vi "AG34980A Get Scan List.vi"(0 "VISA resource name":refnum<visa-resource-name>, 11 "error in (no error)":errorcluster) -> (4 "Channel List":string, 6 "Num of Chans":i32, 15 "error out":errorcluster)   [LabVIEW 2016]
doc: "This VI can be used to query the current scan list size as well as the time that the current scan started."
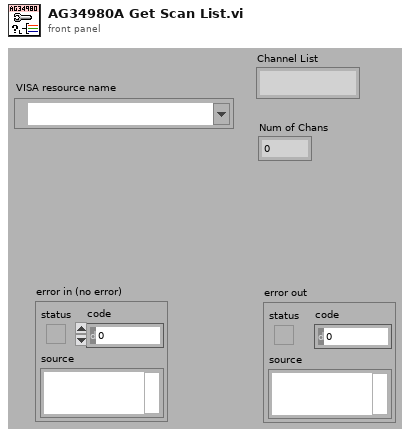
[diagram p1: front panel]
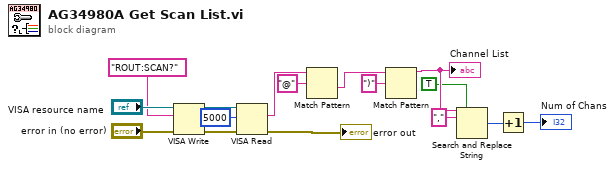
[diagram p0: block diagram]
diagram:
  n1 = VISA Write(VISA resource name="VISA resource name", write buffer="ROUT:SCAN?", error in (no error)="error in (no error)") -> (VISA resource name out=w11:refnum<visa-resource-name>, error out=w12:errorcluster)  [unwired: 1 out]
  n2 = VISA Read(VISA resource name=w11, byte count=u32 5000, error in (no error)=w12) -> (read buffer=w9:string, error out=→"error out":errorcluster)  [unwired: 2 out]
  n3 = Match Pattern(string=w9, regular expression="@") -> (after substring=w7:string)  [unwired: 1 in, 3 out]
  n4 = Match Pattern(string=w7, regular expression=")") -> (before substring=w5:string)  [unwired: 1 in, 3 out]
  "Channel List" <- w5
  n5 = Search and Replace String(replace all?=TRUE ("replace all? (F)"), input string=w5, search string=",") -> (number of replacements=w2:i32)  [unwired: 5 in, 3 out]
  n6 = Increment(x=w2) -> (x+1=→"Num of Chans":i32)
